vi "set_LM_ID.vi"(8 "error in (no error)":errorcluster caption="错误输入（无错误）", 10 "LM ID":T1=1 items=["none", "S1", "S2", "S3"], 11 "LimitSwitch输入":refnum<class "LimitSwitch.lvclass">) -> (0 "error out":errorcluster caption="错误输出", 3 "LimitSwitch输出":refnum<class "LimitSwitch.lvclass">)   [LabVIEW 2016, in "MotionControl.lvlib" / "LimitSwitch.lvclass"]
uses:
  <userlib>/MotionControl/LimitSwitch/LimitSwitch.lvclass
  <userlib>/MotionControl/LimitSwitch/LM_ID.ctl
  <userlib>/MotionControl/LimitSwitch/LimitSwitch.lvclass/LimitSwitch.ctl
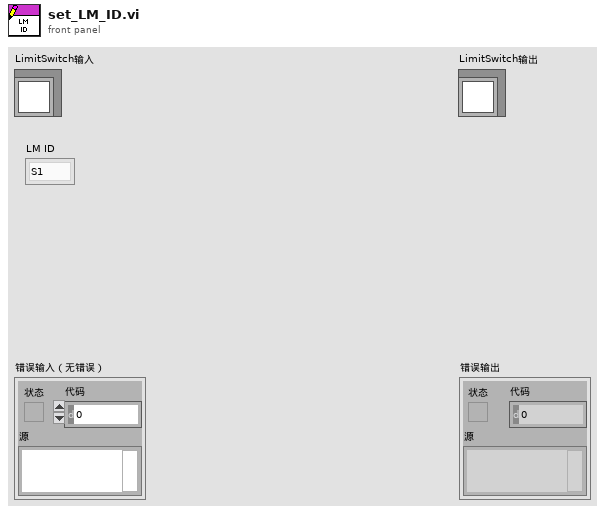
[diagram p1: front panel]
types:
  T1 = typedef "MotionControl.lvlib/LimitSwitch.lvclass/LM_ID.ctl" = i32
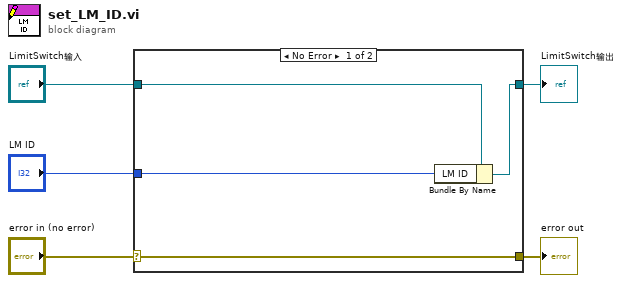
[diagram p0: block diagram]
diagram:
  n1 = case shown="No Error" "error in (no error)" {
    selector: "error in (no error)" -> [w9 w10]
    tunnel: [w9 w10] -> w4
    tunnel: [w7 w11] -> w2
    tunnel: "LimitSwitch输入" -> [w8 w11]
    tunnel: "LM ID" -> [w6 _]
    frame No Error {
      n2 = Bundle By Name(cluster=w8, "LM ID"=w6) -> (w7:refnum<class "LimitSwitch.lvclass">)
    }
    frame Error {
    }
  }
  "error out" <- w4
  "LimitSwitch输出" <- w2
